vi "DLL Library Path VIs.vi"() -> (0 "OCTNumerics":path, 1 "Alazar":path, 2 "GPU FFT birefringence simple ret":path, 3 "SpectralRadarDLL":path, 9 "GPU FFT birefringence":path, 10 "GPU FFT amp phase":path, 11 "GPU FFT amplitude":path)   [LabVIEW 2018]
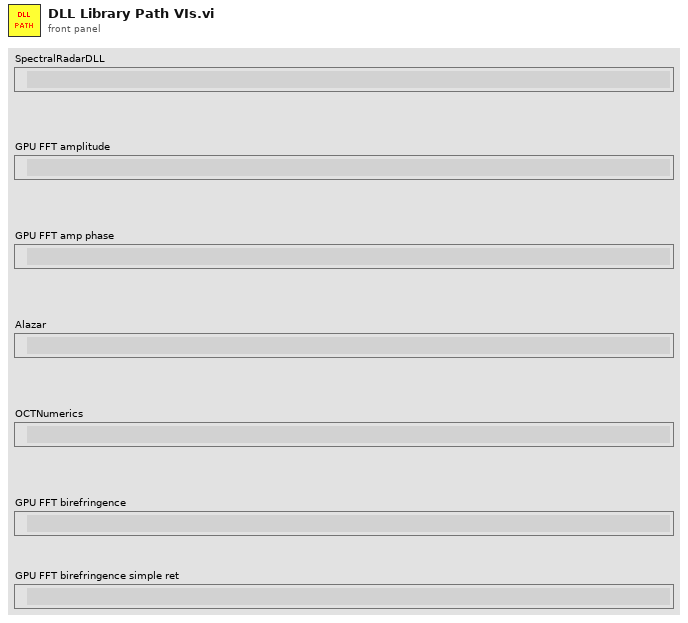
[diagram p1: front panel]
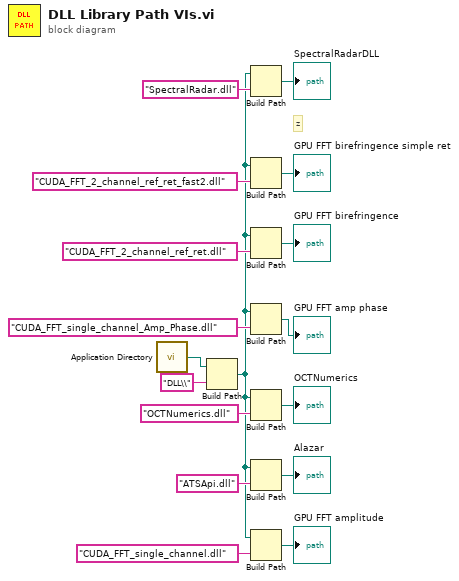
[diagram p0: block diagram]
diagram:
  # "z"
  n1 = call <vilib>:"Application Directory.vi"() -> ("Application Directory"=w17:path)
  n2 = Build Path(base path=w17, name or relative path="DLL\\") -> (appended path=w1:path)
  n3 = Build Path(base path=w1, name or relative path="SpectralRadar.dll") -> (appended path=→"SpectralRadarDLL":path)
  n4 = Build Path(base path=w1, name or relative path="CUDA_FFT_2_channel_ref_ret_fast2.dll") -> (appended path=→"GPU FFT birefringence simple ret":path)
  n5 = Build Path(base path=w1, name or relative path="CUDA_FFT_2_channel_ref_ret.dll") -> (appended path=→"GPU FFT birefringence":path)
  n6 = Build Path(base path=w1, name or relative path="CUDA_FFT_single_channel_Amp_Phase.dll") -> (appended path=→"GPU FFT amp phase":path)
  n7 = Build Path(base path=w1, name or relative path="OCTNumerics.dll") -> (appended path=→"OCTNumerics":path)
  n8 = Build Path(base path=w1, name or relative path="ATSApi.dll") -> (appended path=→"Alazar":path)
  n9 = Build Path(base path=w1, name or relative path="CUDA_FFT_single_channel.dll") -> (appended path=→"GPU FFT amplitude":path)
